vi "Get Length.vi"(3 "Error In":errorcluster, 5 "object in":refnum<class "Stack.lvclass">) -> (0 "Error Out":errorcluster, 1 "Length":i32, 2 "object out":refnum<class "Stack.lvclass">)   [LabVIEW 2024, in "Stack.lvclass"]
uses:
  Stack.lvclass
  Stack.lvclass/Stack.ctl
panel:
  # "Connector Pane"
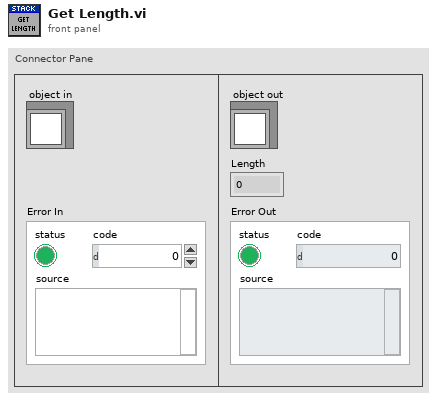
[diagram p1: front panel]
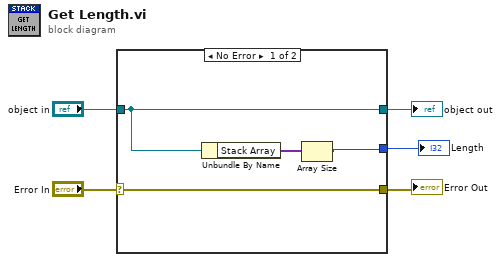
[diagram p0: block diagram]
diagram:
  n1 = case shown="No Error" "Error In" {
    selector: "Error In" -> [w9 w11]
    tunnel: [w9 w11] -> w4
    tunnel: [w8 w10] -> w2
    tunnel: "object in" -> [w8 w10]
    tunnel: [w6 _] -> w1
    frame No Error {
      n2 = Unbundle By Name(w8) -> ("Stack Array"=w7:variant[])
      n3 = Array Size(array=w7) -> (size(s)=w6:i32)
    }
    frame Error {
    }
  }
  "Error Out" <- w4
  "object out" <- w2
  "Length" <- w1
